vi "WS_Main.vi"(6 "LabVIEW Web Service":refnum<class "Web Service.lvclass">) -> ()   [LabVIEW 2016]
uses:
  <vilib>/wsapi/Web Service.lvclass
  Libraries/WSsupport/GV_Repos.vi
  Libraries/WSsupport/WSsupport.lvlib
  Libraries/Packages/VIPM/VIPM.lvlib
  Libraries/Packages/GPM/GPM.lvlib
panel:
  # "Use the web service input terminal to call the VIs on the Service subpalette of the Web Services palette. Do not remove it from the connector pane unless you don't need access to the palette."
  # "Any additional terminals added to the connector pane of a startup VI will be ignored."
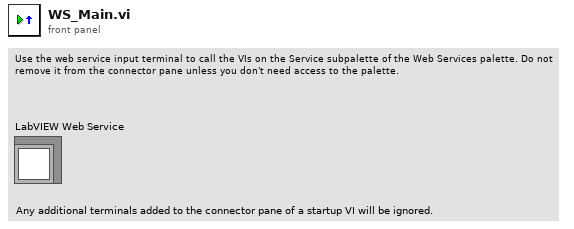
[diagram p1: front panel]
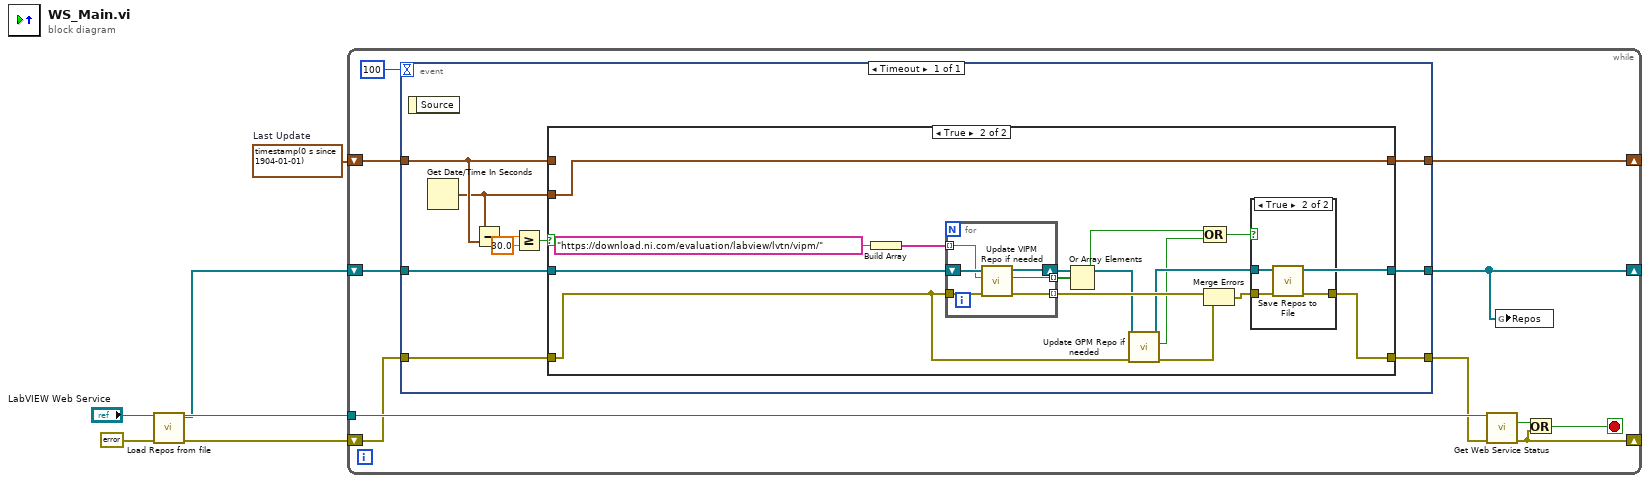
[diagram p0: block diagram]
diagram:
  w3 = timestamp(0 s since 1904-01-01)  # Last Update
  n1 = call "Load Repos from file.vi"("error in"=errorcluster {"status"=FALSE, "code"=0, "source"=""} ("error constant")) -> ("error out"=w2:errorcluster, "Repos"=w1:refnum<class "Repo.lvclass">[])  [unwired: 9 in]
  n2 = while {
    tunnel: "LabVIEW Web Service" -> [w15]
    shift-right: [w13] -> _
    shift-left: w2 -> [w7]
    shift-right: [w11] -> _
    shift-left: w3 -> [w10]
    shift-right: [w8] -> _
    shift-left: w1 -> [w9]
    stop <- w14 stop-if-true
    # "Add processing code here. The loop will terminate on error or when the web service stops. If the loop performs long-running operations, consider adding additional Get Web Service Status calls to cancel those operations."
    n3 = event shown="[0] Timeout" {
      selector: _ -> [_]
      dyn-events: _ -> [_]
      timeout: 100 -> [_]
      tunnel: [w19] -> w11
      tunnel: w10 -> [w18]
      tunnel: w9 -> [w23]
      tunnel: [w22] -> w8
      tunnel: [w21] -> w6
      tunnel: w7 -> [w20]
      event Timeout {
        n4 = event-data() -> ()  [unwired: 1 in, 1 out]
        n5 = Get Date/Time In Seconds() -> (seconds since 1Jan1904=w17:timestamp)
        n6 = Subtract(x=w17, y=w18) -> (x-y=w26:dbl)
        n7 = Greater Or Equal?(x=w26, y=30.0) -> (x >= y?=w24:bool)
        n8 = case shown="True" w24 {
          tunnel: w23 -> [w29 w44]
          tunnel: [w29 w34] -> w22
          tunnel: [w28 w39] -> w21
          tunnel: w20 -> [w28 w33]
          tunnel: [w27 w36] -> w19
          tunnel: w18 -> [w27 _]
          tunnel: w17 -> [_ w36]
          frame False {
          }
          frame True {
            n9 = Build Array("https://download.ni.com/evaluation/labview/lvtn/vipm/" ("Repo URL")) -> (w42:string[])
            n10 = for {
              shift-right: [w53] -> w38
              shift-left: w44 -> [w54]
              tunnel: w42 -> [w52] mode=indexing
              tunnel: [w49] -> w40 mode=indexing
              tunnel: w33 -> [w51]
              tunnel: [w50] -> w41 mode=indexing
              n11 = call "Update VIPM Repo if needed.vi"("error in (no error)"=w51, "Repo URL"=w52, "Repos in"=w54) -> ("error out"=w50:errorcluster, "Updated?"=w49:bool, "Repos out"=w53:refnum<class "Repo.lvclass">[])  [unwired: 6 in]
            }
            n12 = Or Array Elements(Boolean array=w40) -> (logical OR=w37:bool)
            n13 = call "Update GPM Repo if needed.vi"("error in (no error)"=w33, "Repos in"=w38) -> ("error out"=w32:errorcluster, "Updated?"=w30:bool, "Repos out"=w34:refnum<class "Repo.lvclass">[])  [unwired: 7 in]
            n14 = Compound Arithmetic op=OR(w37, w30) -> (w31:bool)
            n15 = Merge Errors(w41, w32) -> (w35:errorcluster)
            n16 = case shown="True" w31 {
              tunnel: w35 -> [w45 w48]
              tunnel: [w45 w47] -> w39
              tunnel: w34 -> [_ w46]
              frame False {
              }
              frame True {
                n17 = call "Save Repos to File.vi"("error in"=w48, "Repos"=w46) -> ("error out"=w47:errorcluster)  [unwired: 9 in]
              }
            }
          }
        }
      }
    }
    n18 = call <vilib>:"Get Web Service Status.vi"("LabVIEW Web Service"=w15, "error in (no error)"=w6) -> ("service stopping?"=w16:bool, "error out"=w13:errorcluster)  [unwired: 11 in, 1 out]
    n19 = global write "GV_Repos.vi" "Repos"(w8) -> ()
    n20 = Or(x=w16, y=w13) -> (x .or. y?=w14:bool)
  }
